vi "Table-Replace subset (start at 00).vi"(8 "error in (no error)":errorcluster, 10 "Table to replace with":string[][](array[string]), 11 "Original table":string[][](array[string])) -> (0 "error out":errorcluster, 3 "Table out":string[][](array[string]))   [LabVIEW 2013]
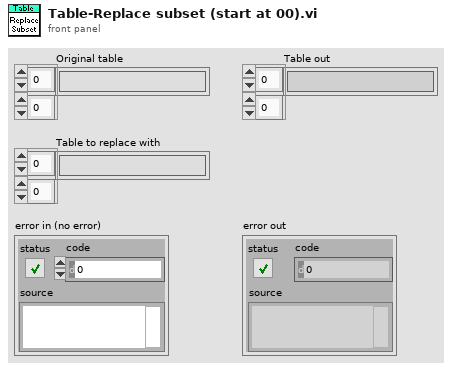
[diagram p1: front panel]
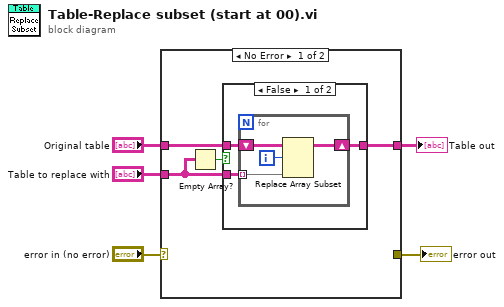
[diagram p0: block diagram]
diagram:
  n1 = case shown="No Error" "error in (no error)" {
    selector: "error in (no error)" -> [_ w18]
    tunnel: [w9 _] -> w5
    tunnel: "Table to replace with" -> [w7 _]
    tunnel: "Original table" -> [w6 _]
    tunnel: [_ w18] -> w1
    frame No Error {
      n2 = Empty Array?(array=w7) -> (empty?=w8:bool)
      n3 = case shown="False" w8 {
        tunnel: w6 -> [w12 w17]
        tunnel: w7 -> [w11 _]
        tunnel: [w10 w17] -> w9
        frame False {
          n4 = for {
            shift-right: [w13] -> w10
            shift-left: w12 -> [w16]
            tunnel: w11 -> [w14] mode=indexing
            i -> [w15]
            n5 = Replace Array Subset(array=w16, new element=w14, index (row)=w15) -> (w13:string[][])  [unwired: 1 in]
          }
        }
        frame True {
        }
      }
    }
    frame Error {
    }
  }
  "Table out" <- w5
  "error out" <- w1
